vi "Wrap Pinmap.vi"(8 "error in":errorcluster, 10 "DUT pin":string, 11 "measurement context in":refnum<class "Measure Call Context.lvclass">) -> (0 "error out":errorcluster, 1 "Channel":string, 2 "session reservation out":refnum<class "Session Reservation.lvclass">, 3 "measurement context out":refnum<class "Measure Call Context.lvclass">)   [LabVIEW 2025, in "Automotive Vision.lvclass"]
uses:
  <vilib>/Plug-In SDKs/Measurements/Measure Call Context/Measure Call Context.lvclass
  <vilib>/Plug-In SDKs/Clients/Session Management V1/Session Reservation/Session Reservation.lvclass
  Automotive Vision.lvclass
  Automotive Vision.lvclass/Automotive Vision.ctl
  <vilib>/Plug-In SDKs/Measurements/Measure Call Context/Reserve Sessions - 1Pin.vi
  session-management/flexrio148x/Session Management flexrio 148x.lvlib
  <vilib>/Plug-In SDKs/Clients/Session Management V1/Session Reservation/Connection.ctl
  session-management/flexrio148x/Connection with Session.ctl
panel:
  out "connection":T1
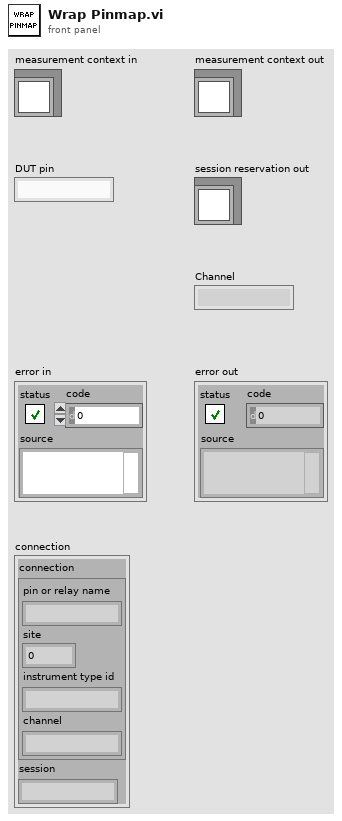
[diagram p1: front panel]
types:
  T1 = typedef "Session Management flexrio 148x.lvlib/Connection with Session.ctl" = cluster{"connection":T2, "session":string}
  T2 = typedef "NI Session Management V1 Client.lvlib/Session Reservation.lvclass/Connection.ctl" = cluster{"pin or relay name":string, "site":i32, "instrument type id":string, "channel":string}
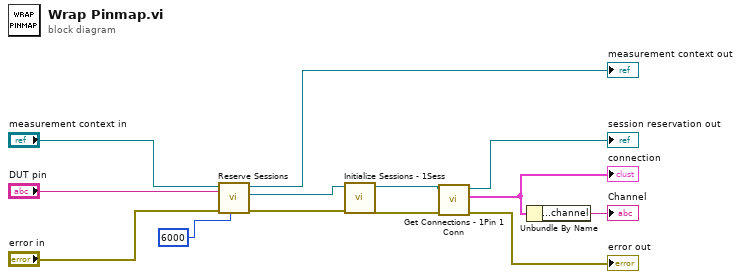
[diagram p0: block diagram]
diagram:
  n1 = call-poly <vilib>:"Reserve Sessions.vi"("timeout (ms)"=6000, "error in"="error in", "pin or relay name"="DUT pin", "measurement context in"="measurement context in") -> ("error out"=w10:errorcluster, "session reservation out"=w9:refnum<class "Session Reservation.lvclass">, "measurement context out"=→"measurement context out":refnum<class "Measure Call Context.lvclass">)  [unwired: 5 in]
  n2 = call "Initialize Sessions - 1Sess.vi"("error in"=w10, "session reservation in"=w9) -> ("error out"=w7:errorcluster, "session reservation out"=w5:refnum<class "Session Reservation.lvclass">)  [unwired: 6 in, 2 out]
  n3 = call "Get Connections - 1Pin 1 Conn.vi"("error in"=w7, "session reservation in"=w5) -> ("error out"=→"error out":errorcluster, "connection"=w2:T1, "session reservation out"=→"session reservation out":refnum<class "Session Reservation.lvclass">)  [unwired: 7 in]
  "connection" <- w2
  n4 = Unbundle By Name(w2) -> ("connection.channel"=→"Channel":string)
